vi "WriteText.vi"(8 "error in (no error)":errorcluster caption="错误输入（无错误）", 10 "Text":refnum<user-event>, 11 "zsActor输入":refnum<class "ActorWrapper.lvclass">) -> (0 "error out":errorcluster caption="错误输出", 3 "zsActor输出":refnum<class "ActorWrapper.lvclass">)   [LabVIEW 2014, in "Wrapper.lvlib" / "ActorWrapper.lvclass"]
uses:
  ActorWrapper.lvclass
  ActorWrapper.lvclass/ActorWrapper.ctl
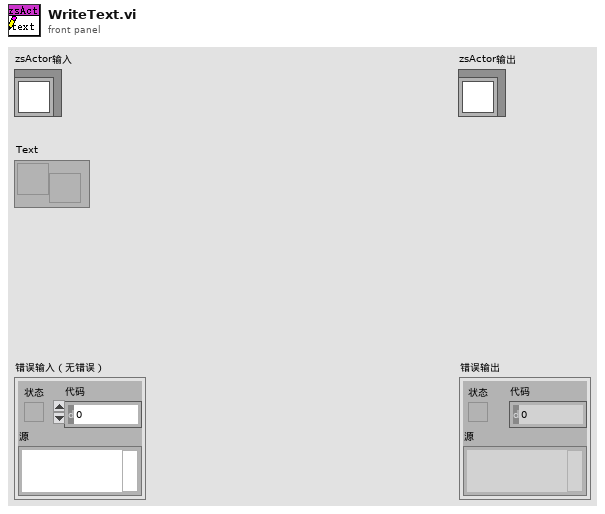
[diagram p1: front panel]
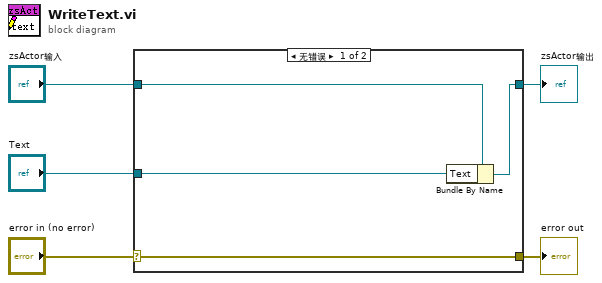
[diagram p0: block diagram]
diagram:
  n1 = case shown="无错误" "error in (no error)" {
    selector: "error in (no error)" -> [w9 w10]
    tunnel: [w9 w10] -> w4
    tunnel: [w7 w11] -> w2
    tunnel: "zsActor输入" -> [w8 w11]
    tunnel: "Text" -> [w6 _]
    frame No Error {
      n2 = Bundle By Name(cluster=w8, "Text"=w6) -> (w7:refnum<class "ActorWrapper.lvclass">)
    }
    frame Error {
    }
  }
  "error out" <- w4
  "zsActor输出" <- w2
